vi "XY点至极坐标点和复数点(标量）.vi"(8 "Error In":errorcluster caption="错误输入", 11 "点":T2 caption="点（双精度）") -> (0 "Error Out":errorcluster caption="错误输出", 2 "复数点":cdb, 3 "极坐标点":T1)   [LabVIEW 2012, in "几何工具.lvlib"]
uses:
  <vilib>/Utility/miscctls.llb/LVPointDoubleTypeDef.ctl
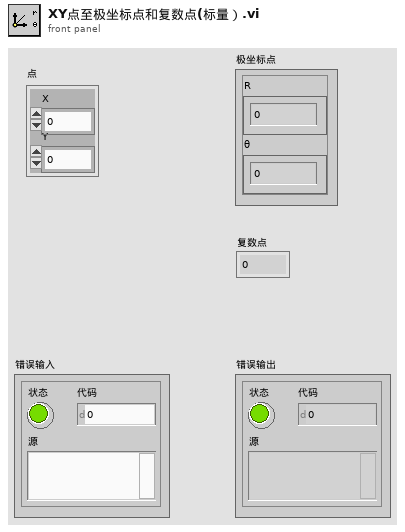
[diagram p1: front panel]
types:
  T1 = typedef "几何工具.lvlib/极坐标.ctl" = cluster{"R":dbl, "θ":dbl}
  T2 = typedef "LVPointDoubleTypeDef.ctl" = cluster{"X":dbl, "Y":dbl}
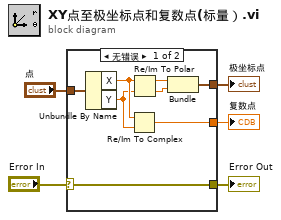
[diagram p0: block diagram]
diagram:
  n1 = case shown="无错误" "Error In" {
    selector: "Error In" -> [w13 w14]
    tunnel: [w13 w14] -> w4
    tunnel: "点" -> [w12 _]
    tunnel: [w9 _] -> w2
    tunnel: [w6 _] -> w1
    frame No Error {
      n2 = Unbundle By Name(w12) -> ("X"=w8:dbl, "Y"=w7:dbl)
      n3 = Re/Im To Complex(1:w7, 2:w8) -> (0:w6:cdb)
      n4 = Re/Im To Polar(2:w7, 3:w8) -> (0:w10:dbl, 1:w11:dbl)
      n5 = Bundle(w11, w10) -> (w9:cluster{dbl, dbl})  [unwired: 1 in]
    }
    frame Error {
    }
  }
  "极坐标点" <- w2
  "Error Out" <- w4
  "复数点" <- w1
